vi "Cancel Task.vi"(8 "error in (no error)":errorcluster, 11 "HttpResponseMessage in":refnum<class "HttpResponseMessage.lvclass">) -> (0 "error out":errorcluster, 3 "HttpResponseMessage out":refnum<class "HttpResponseMessage.lvclass">)   [LabVIEW 2018, in "LabVIEWHTTPClient_NET.lvlib" / "HttpResponseMessage.lvclass"]
uses:
  HttpResponseMessage.lvclass
  HttpResponseMessage.lvclass/HttpResponseMessage.ctl
  Accessors/Read NET_CancellationSource.vi
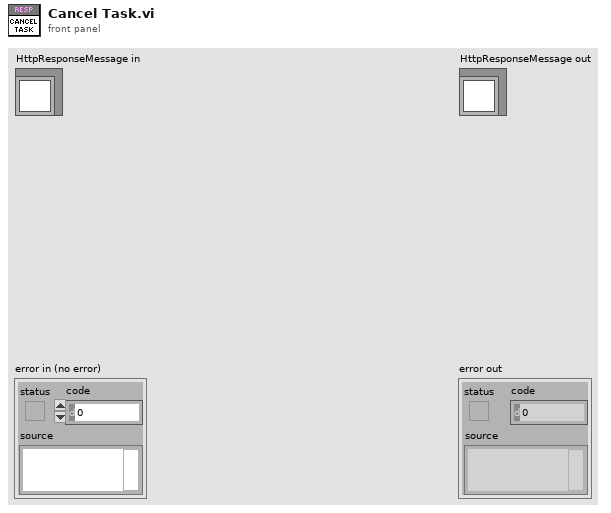
[diagram p1: front panel]
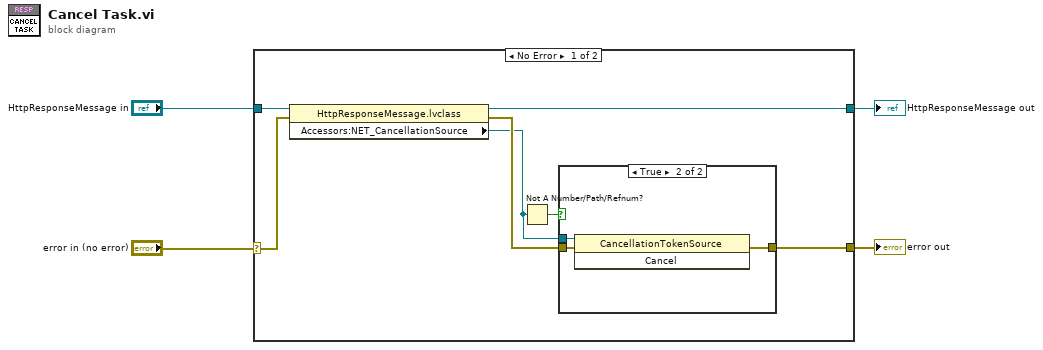
[diagram p0: block diagram]
diagram:
  n1 = case shown="No Error" "error in (no error)" {
    selector: "error in (no error)" -> [w11 w17]
    tunnel: [w5 w17] -> w3
    tunnel: [w9 w16] -> w1
    tunnel: "HttpResponseMessage in" -> [w10 w16]
    frame No Error {
      n2 = property class="HttpResponseMessage.lvclass"(reference=w10, error in=w11) -> (reference out=w9:refnum<class "HttpResponseMessage.lvclass">, error out=w7:errorcluster, "Accessors:NET_CancellationSource"=w6:refnum<k24>)
      n3 = Not A Number/Path/Refnum?(number/path/refnum=w6) -> (NaN/Path/Refnum?=w8:bool)
      n4 = case shown="True" w8 {
        tunnel: w7 -> [w12 w14]
        tunnel: w6 -> [_ w15]
        tunnel: [w12 w13] -> w5
        frame False {
        }
        frame True {
          n5 = invoke class="CancellationTokenSource" method="Cancel"(reference=w15, error in=w14) -> (error out=w13:errorcluster)  [unwired: 1 in, 2 out]
        }
      }
    }
    frame Error {
    }
  }
  "error out" <- w3
  "HttpResponseMessage out" <- w1
